vi "Refresh UI.vi"(11 "references":T1) -> (0 "error out":errorcluster)   [LabVIEW 2013, in "tag bus configurable plugin editor node.lvclass"]
uses:
  tag bus configurable plugin editor node.lvclass
  <vilib>/NI/DCAF Table API/Table Manager/object ref.ctl
  <vilib>/NI/Tag Bus Data Framework/Configuration Editor/Classes/Engine Parent/Engine Parent Editor Node.lvclass
  <vilib>/NI/Tag Bus Data Framework/Configuration Editor/Classes/Module editor node/module editor node.lvclass
  <vilib>/NI/DCAF Table API/Table Manager/Table Manager.lvclass
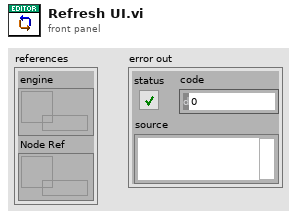
[diagram p1: front panel]
types:
  T1 = typedef "Table Manager.lvlib/Table Manager.lvclass/object ref.ctl" = cluster{"engine":refnum<data-value>, "Node Ref":refnum<data-value>}
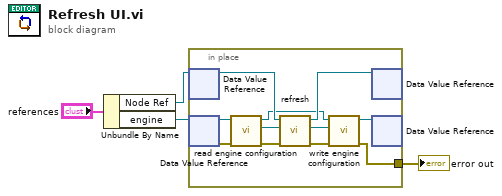
[diagram p0: block diagram]
diagram:
  n1 = Unbundle By Name("references") -> ("Node Ref"=w2:refnum<data-value>, "engine"=w3:refnum<data-value>)
  n2 = in-place {
    in-place-border: [w7] -> w4
    n3 = in-place-dvr #1(w2) -> (w15:refnum<class "module editor node.lvclass">)  [unwired: 1 out]
    n4 = in-place-dvr #2(w3) -> (w13:refnum<class "Engine Parent Editor Node.lvclass">, w12:errorcluster)
    n5 = call <vilib>:"read engine configuration.vi"("error in"=w12, "Engine Parent Editor Node in"=w13) -> ("error out"=w11:errorcluster, "engine configuration"=w10:refnum<class "engine configuration.lvclass">, "Engine Parent Editor Node out"=w5:refnum<class "Engine Parent Editor Node.lvclass">)  [unwired: 7 in]
    n6 = call-dynamic "refresh.vi"("error in (no error)"=w11, "Engine Configuration In"=w10, "Module Editor Node In"=w15) -> ("error out"=w8:errorcluster, "Engine Configuration Out"=w9:refnum<class "engine configuration.lvclass">, "Module Editor Node Out"=w14:refnum<class "module editor node.lvclass">)  [unwired: 6 in]
    n7 = call <vilib>:"write engine configuration.vi"("error in"=w8, "engine configuration"=w9, "Engine Parent Editor Node in"=w5) -> ("error out"=w7:errorcluster, "Engine Parent Editor Node out"=w6:refnum<class "Engine Parent Editor Node.lvclass">)  [unwired: 7 in]
    n8 = in-place-dvr #1(w14) -> ()  [unwired: 2 out]
    n9 = in-place-dvr #2(w6) -> ()  [unwired: 2 out]
  }
  "error out" <- w4
